vi "DecodeFlowUnit SubVI.vi"(1 "FlowUnit":u8) -> (0 "Flow Unit Comment":string)   [LabVIEW 2019]
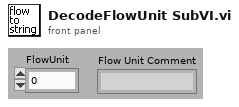
[diagram p1: front panel]
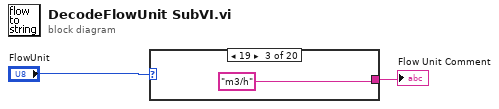
[diagram p0: block diagram]
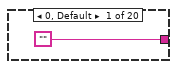
[diagram p2: hidden frame]
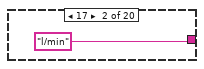
[diagram p3: hidden frame]
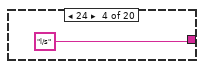
[diagram p4: hidden frame]
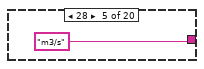
[diagram p5: hidden frame]
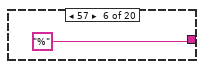
[diagram p6: hidden frame]
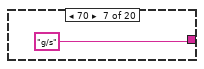
[diagram p7: hidden frame]
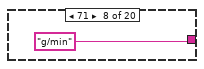
[diagram p8: hidden frame]
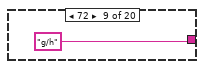
[diagram p9: hidden frame]
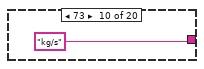
[diagram p10: hidden frame]
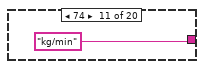
[diagram p11: hidden frame]
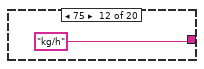
[diagram p12: hidden frame]
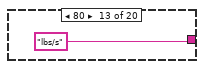
[diagram p13: hidden frame]
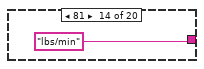
[diagram p14: hidden frame]
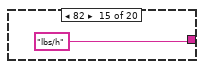
[diagram p15: hidden frame]
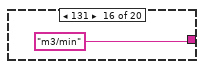
[diagram p16: hidden frame]
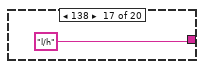
[diagram p17: hidden frame]
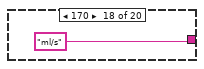
[diagram p18: hidden frame]
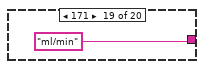
[diagram p19: hidden frame]
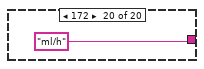
[diagram p20: hidden frame]
diagram:
  n1 = case shown="19" "FlowUnit" {
    tunnel: ["" "l/min" "m3/h" "l/s" "m3/s" "%" "g/s" "g/min" "g/h" "kg/s" "kg/min" "kg/h" "lbs/s" "lbs/min" "lbs/h" "m3/min" "l/h" "ml/s" "ml/min" "ml/h"] -> w2
    frame 0, Default {
    }
    frame 17 {
    }
    frame 19 {
    }
    frame 24 {
    }
    frame 28 {
    }
    frame 57 {
    }
    frame 70 {
    }
    frame 71 {
    }
    frame 72 {
    }
    frame 73 {
    }
    frame 74 {
    }
    frame 75 {
    }
    frame 80 {
    }
    frame 81 {
    }
    frame 82 {
    }
    frame 131 {
    }
    frame 138 {
    }
    frame 170 {
    }
    frame 171 {
    }
    frame 172 {
    }
  }
  "Flow Unit Comment" <- w2
